vi "Set Tray Icon.vi"   [LabVIEW 2018, in "NotifyIcon.lvclass"]
doc: "This VI is used to set the icon that is associated with the context menu and shown in the notification area.\nThe VI is polymorphic and will accept a string or a path as the source of the data.\n\nIf the source is a string the VI expects the string to be a binary representation of an ICO file. This is usefull because the icon source can be included in the VI code as a constant, thus decreasing the need for external files.\n\nIf the source is a path, the VI will load and resize any BMP, GIF, JPG, PNG, TIFF or ICO file and use the content as the icon.\n\n\nStinus Olsen\nCIM Industrial Systems A/S\n22. Feb. 2011 15:06\nmailto: seo@cim.as"
uses:
  NotifyIcon.lvclass
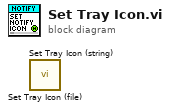
[diagram p0: block diagram]
diagram:
  n1 = call "Set Tray Icon (file).vi"() -> ()  [unwired: 14 in, 2 out]
  n2 = call "Set Tray Icon (string).vi"() -> ()  [unwired: 14 in, 2 out]
